vi "Close.vi"(8 "Error In":errorcluster, 11 "SerialComm in":refnum<class "SerialComm.lvclass">) -> (0 "Error Out":errorcluster, 3 "SerialComm out":refnum<class "SerialComm.lvclass">)   [LabVIEW 2016, in "SerialComm.lvclass"]
uses:
  SerialComm.lvclass
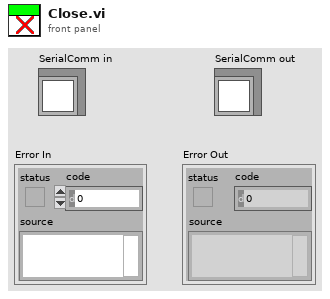
[diagram p1: front panel]
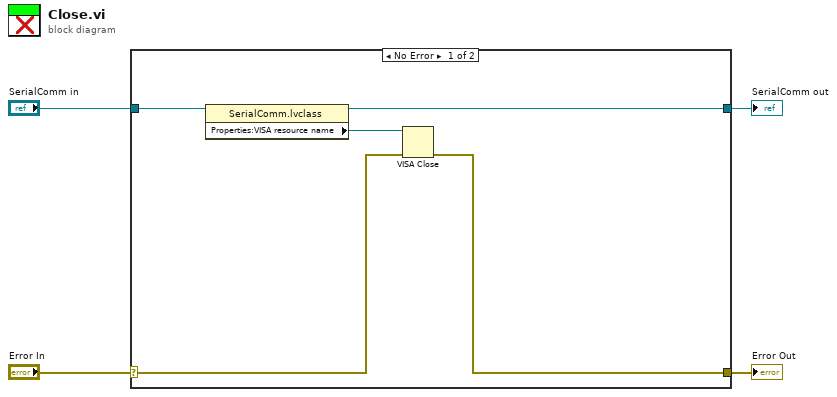
[diagram p0: block diagram]
diagram:
  n1 = case shown="No Error" "Error In" {
    selector: "Error In" -> [w6 w11]
    tunnel: [w5 w11] -> w3
    tunnel: [w8 w10] -> w1
    tunnel: "SerialComm in" -> [w9 w10]
    frame No Error {
      n2 = property class="SerialComm.lvclass"(reference=w9) -> (reference out=w8:refnum<class "SerialComm.lvclass">, "Properties:VISA resource name"=w7:refnum<visa-resource-name>)  [unwired: 1 in, 1 out]
      n3 = VISA Close(VISA resource name=w7, error in (no error)=w6) -> (error out=w5:errorcluster)
    }
    frame Error {
    }
  }
  "Error Out" <- w3
  "SerialComm out" <- w1
